vi "Impedance Spec Limit Line.vi"(0 "Time Array":dbl[](array[numeric]), 1 "Impedance Data":dbl[](array[numeric]), 2 "Impedance Spec String":string="1@110@2@105;1@90@2@95", 4 "Des.":string="TDD11") -> (19 "Test Data":T1, 20 "test passed?":bool=TRUE caption="Test Pass?", 21 "Max  value":dbl[](array[numeric])=[102.14453345181848, 103.42341181521715], 23 "Min value":dbl[](array[numeric])=[99.46210027960517, 101.75922922405344], 24 "Upper Spec":dbl[](array[numeric]), 25 "Lower Spec":dbl[](array[numeric]), 26 "Test Summary":string, 27 "Impedance Chart":T2(graph))   [LabVIEW 2011]
uses:
  <vilib>/measure/mamon.llb/Limit Testing Time.vi
  <vilib>/measure/NI_MAPro.lvlib
panel:
  out "Upper Spec Position":dbl[](array[numeric])=[799.7999860194963, 799.7999860194963, 1199.6999790292443, 1199.6999790292443]
  out "Lower Spec Position":dbl[](array[numeric])=[799.7999860194963, 799.7999860194963, 1199.6999790292443, 1199.6999790292443]
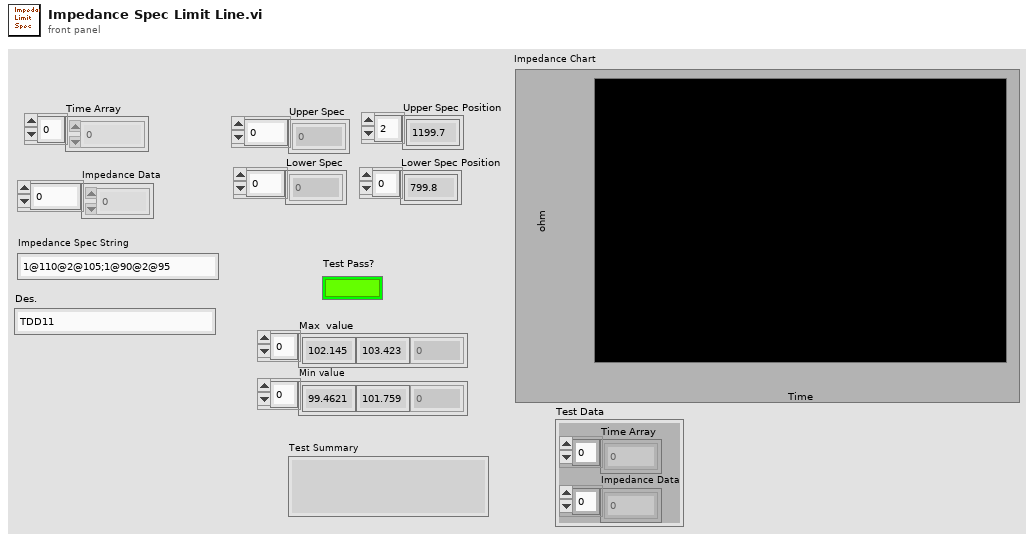
[diagram p1: front panel]
types:
  T1 = cluster{"Time Array":dbl[], "Impedance Data":dbl[]}
  T2 = cluster{"Time Array":dbl[], "Lower Spec":dbl[]}[]
  T3 = cluster{"Time Array":dbl[], "Impedance Data":dbl[]}[]
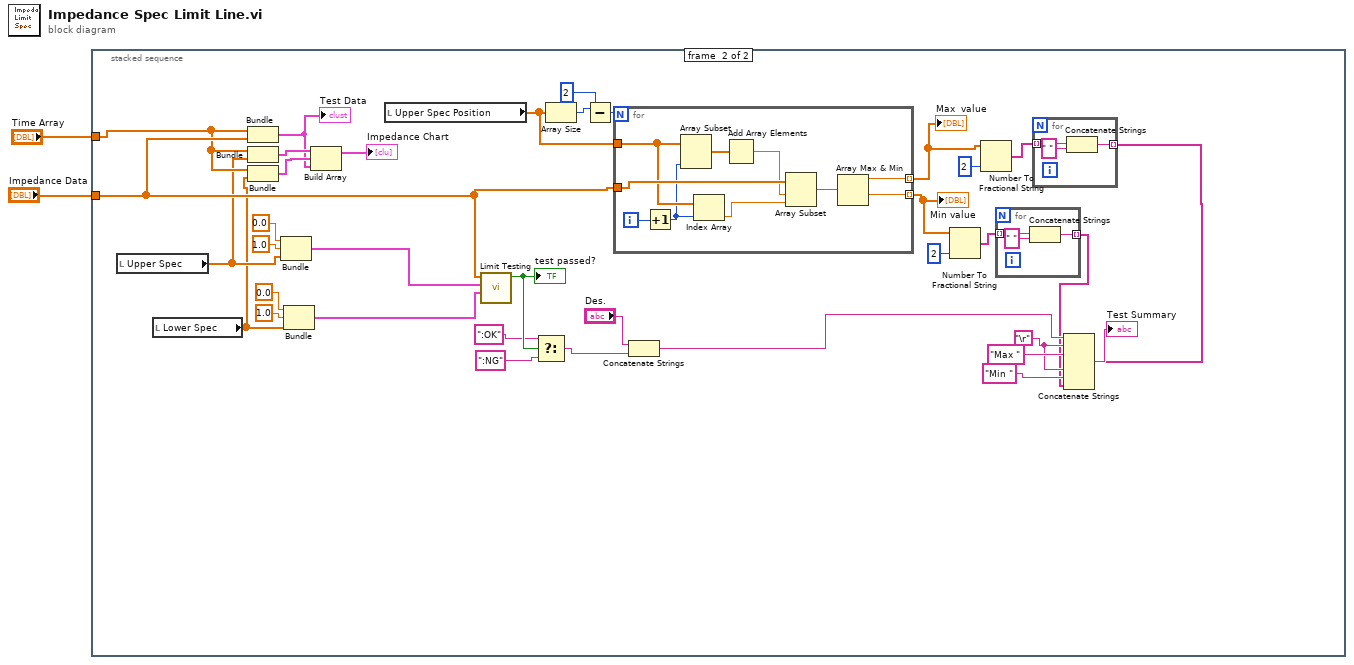
[diagram p0: block diagram]
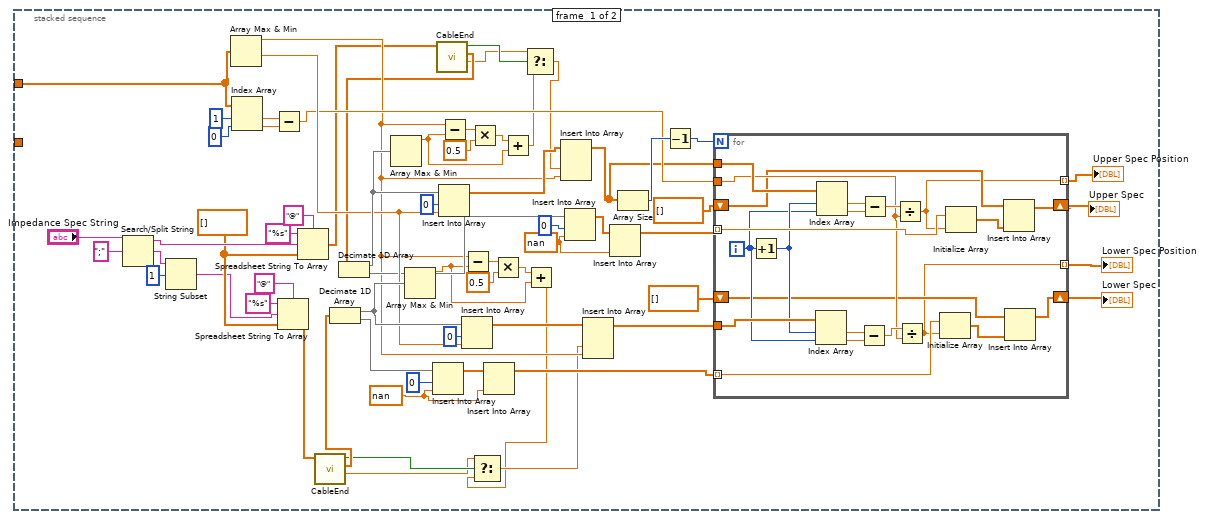
[diagram p2: hidden frame]
diagram:
  n1 = stacked-sequence {
    tunnel: "Time Array" -> [w15 w113]
    tunnel: "Impedance Data" -> [_ w114]
    frame #0 {
      w23 = nan ("新元素/子数组")
      w20 = nan ("新元素/子数组")
      w58 = dbl[] []
      n2 = Search/Split String(string="Impedance Spec String", search string/char (-)=";" ("搜索字符串/字符(-)")) -> (substring before match=w63:string, match + rest of string=w65:string)  [unwired: 1 in, 1 out]
      n3 = String Subset(string=w65, offset (0)=1 ("偏移量(0)")) -> (substring=w57:string)  [unwired: 1 in]
      n4 = Array Max & Min(array=w15) -> (max value=w25:dbl, min value=w40:dbl)  [unwired: 2 out]
      n5 = Index Array(array=w15, index #1=1 ("索引"), index #2=0 ("索引")) -> (element #1=w54:dbl, element #2=w53:dbl)
      n6 = Subtract(x=w54, y=w53) -> (x-y=w37:dbl)
      n7 = Spreadsheet String To Array(delimiter (Tab)="@" ("分隔符(Tab)"), format string="%s" ("格式字符串"), spreadsheet string=w57, array type (2D Dbl)=w58) -> (array=w14:dbl[])
      n8 = Spreadsheet String To Array(delimiter (Tab)="@" ("分隔符(Tab)"), format string="%s" ("格式字符串"), spreadsheet string=w63, array type (2D Dbl)=w58) -> (array=w8:dbl[])
      n9 = call "CableEnd.vi"("Raw"=w14) -> ("CableEnd"=w11:dbl, "Filtered"=w13:dbl[], "CableEndSet"=w12:bool)  [unwired: 8 in]
      n10 = Decimate 1D Array(w13) -> (w41:dbl[], w33:dbl[])
      n11 = Array Max & Min(array=w41) -> (max value=w27:dbl)  [unwired: 3 out]
      n12 = Insert Into Array(array=w33, index=0 ("索引"), new element=w23) -> (w24:dbl[])
      n13 = call "CableEnd.vi"("Raw"=w8) -> ("CableEnd"=w5:dbl, "Filtered"=w7:dbl[], "CableEndSet"=w6:bool)  [unwired: 8 in]
      n14 = Decimate 1D Array(w7) -> (w51:dbl[], w35:dbl[])
      n15 = Array Max & Min(array=w51) -> (max value=w26:dbl)  [unwired: 3 out]
      n16 = Insert Into Array(array=w51, index=0 ("索引"), new element=w40) -> (w48:dbl[])
      n17 = Subtract(x=w25, y=w26) -> (x-y=w50:dbl)
      n18 = Insert Into Array(array=w41, index=0 ("索引"), new element=w40) -> (w45:dbl[])
      n19 = Subtract(x=w25, y=w27) -> (x-y=w43:dbl)
      n20 = Multiply(x=w50, y=0.5) -> (x*y=w47:dbl)
      n21 = Insert Into Array(array=w24, new element=w23) -> (w22:dbl[])  [unwired: 1 in]
      n22 = Multiply(x=w43, y=0.5) -> (x*y=w46:dbl)
      n23 = Add(x=w47, y=w26) -> (x+y=w4:dbl)
      n24 = Select(t=w5, s=w6, f=w4) -> (s? t:f=w3:dbl)
      n25 = Add(x=w46, y=w27) -> (x+y=w9:dbl)
      n26 = Select(t=w11, s=w12, f=w9) -> (s? t:f=w10:dbl)
      n27 = Insert Into Array(array=w48, new element #1=w3, new element #2=w25) -> (w36:dbl[])  [unwired: 1 in]
      n28 = Insert Into Array(array=w35, index=0 ("索引"), new element=w20) -> (w21:dbl[])
      n29 = Insert Into Array(array=w45, new element #1=w10, new element #2=w25) -> (w31:dbl[])  [unwired: 1 in]
      n30 = Insert Into Array(array=w21, new element=w20) -> (w19:dbl[])  [unwired: 1 in]
      n31 = Array Size(array=w36) -> (size(s)=w38:i32)
      n32 = Decrement(x=w38) -> (x-1=w39:i32)
      n33 = for {
        N: w39 -> [_]
        tunnel: w37 -> [w77]
        tunnel: w36 -> [w88]
        tunnel: w19 -> [w84] mode=indexing
        tunnel: w22 -> [w76] mode=indexing
        tunnel: w31 -> [w83]
        shift-right: [w73] -> w18
        shift-left: dbl[] [] -> [w75]
        shift-right: [w70] -> w28
        shift-left: dbl[] [] -> [w71]
        tunnel: [w69] -> w16 mode=indexing
        tunnel: [w68] -> w17 mode=indexing
        i -> [w81]
        n34 = Increment(x=w81) -> (x+1=w82:i32)
        n35 = Index Array(array=w83, index #1=w82, index #2=w81) -> (element #1=w79:dbl, element #2=w80:dbl)
        n36 = Index Array(array=w88, index #1=w82, index #2=w81) -> (element #1=w87:dbl, element #2=w86:dbl)
        n37 = Subtract(x=w79, y=w80) -> (x-y=w78:dbl)
        n38 = Subtract(x=w87, y=w86) -> (x-y=w85:dbl)
        n39 = Divide(x=w85, y=w77) -> (x/y=w69:dbl)
        n40 = Divide(x=w78, y=w77) -> (x/y=w68:dbl)
        n41 = Initialize Array(w76, w68) -> (w72:dbl[])
        n42 = Initialize Array(w84, w69) -> (w74:dbl[])
        n43 = Insert Into Array(array=w75, new element=w74) -> (w73:dbl[])  [unwired: 1 in]
        n44 = Insert Into Array(array=w71, new element=w72) -> (w70:dbl[])  [unwired: 1 in]
      }
      "Lower Spec" <- w28
      "Upper Spec" <- w18
      "Lower Spec Position" <- w17
      "Upper Spec Position" <- w16
    }
    frame #1 {
      w98 = "\r"
      n45 = local read "Upper Spec"() -> (w112:dbl[])
      n46 = local read "Lower Spec"() -> (w111:dbl[])
      n47 = Bundle("Time Array"=w113, "Impedance Data"=w114) -> (w89:T1)  [unwired: 1 in]
      "Test Data" <- w89
      n48 = Bundle("Time Array"=w113, "Upper Spec"=w112) -> (w110:cluster{"Time Array":dbl[], "Upper Spec":dbl[]})  [unwired: 1 in]
      n49 = Bundle("Time Array"=w113, "Lower Spec"=w111) -> (w109:cluster{"Time Array":dbl[], "Lower Spec":dbl[]})  [unwired: 1 in]
      n50 = Bundle("x0"=0.0, "dx"=1.0, "Upper Spec"=w112) -> (w119:cluster{"x0":dbl, "dx":dbl, "Upper Spec":dbl[]})  [unwired: 1 in]
      n51 = Bundle("x0"=0.0, "dx"=1.0, "Lower Spec"=w111) -> (w120:cluster{"x0":dbl, "dx":dbl, "Lower Spec":dbl[]})  [unwired: 1 in]
      n52 = Build Array(w110, w109, w89) -> (→"Impedance Chart":T3)
      n53 = local read "Upper Spec Position"() -> (w115:dbl[])
      n54 = call-poly <vilib>:"Limit Testing.vi"("lower limit"=w120, "upper limit"=w119, "signal in"=w114) -> ("test passed?"=w107:bool)  [unwired: 3 in, 5 out]
      "test passed?" <- w107
      n55 = Select(t=":OK" ("Des."), s=w107, f=":NG" ("Des.")) -> (s? t:f=w99:string)
      n56 = Array Size(array=w115) -> (size(s)=w117:i32)
      n57 = Subtract(x=w117, y=2) -> (x-y=w118:i32)
      n58 = for {
        N: w118 -> [_]
        tunnel: w115 -> [w138]
        tunnel: w114 -> [w139]
        tunnel: [w132] -> w95 mode=indexing
        tunnel: [w131] -> w92 mode=indexing
        i -> [w137]
        n59 = Increment(x=w137) -> (x+1=w135:i32)
        n60 = Array Subset(array=w138, length=w135) -> (w140:dbl[])  [unwired: 1 in]
        n61 = Index Array(array=w138, index=w135) -> (element=w134:dbl)
        n62 = Add Array Elements(numeric array=w140) -> (sum=w136:dbl)
        n63 = Array Subset(array=w139, index=w136, length=w134) -> (w133:dbl[])
        n64 = Array Max & Min(array=w133) -> (max value=w132:dbl, min value=w131:dbl)  [unwired: 2 out]
      }
      "Max  value" <- w95
      "Min value" <- w92
      n65 = Concatenate Strings("Des.", w99) -> (w96:string)
      n66 = Number To Fractional String(number=w92, precision (6)=i16 2 ("精度(6)")) -> (F-format string=w91:string[])  [unwired: 2 in]
      n67 = Number To Fractional String(number=w95, precision (6)=i16 2 ("精度(6)")) -> (F-format string=w94:string[])  [unwired: 2 in]
      n68 = for {
        tunnel: w91 -> [w127] mode=indexing
        tunnel: [w125] -> w90 mode=indexing
        n69 = Concatenate Strings(w127, " " ("字符串")) -> (w125:string)
      }
      n70 = for {
        tunnel: w94 -> [w130] mode=indexing
        tunnel: [w128] -> w93 mode=indexing
        n71 = Concatenate Strings(w130, " " ("字符串")) -> (w128:string)
      }
      n72 = Concatenate Strings(w96, w98, "Max " ("字符串"), w93, w98, "Min " ("字符串"), w90) -> (→"Test Summary":string)
    }
  }
